vi "BPCS-Malicious-DE-OnePID.vi"() -> ()   [LabVIEW 2017]
uses:
  <vilib>/Platform/TimedLoop/XDataNode/timing_clust.ctl
  <vilib>/Platform/TimedLoop/XDataNode/nitl_modes.ctl
  <vilib>/Platform/TimedLoop/XDataNode/wakeup.ctl
  <vilib>/addons/control/pid/pid.llb/PID Advanced (DBL).vi
  <vilib>/Platform/TimedLoop/XDataNode/XDataNode.xnode
  <vilib>/Platform/TimedLoop/XDataNode/XDNodeRunTimeDep.lvlib
  <vilib>/addons/control/pid/NI_PID_pid.lvlib
panel:
  out "Finished Late? [i-1]":bool
  out "Actual End [i-1]":i64
  out "Expected End [i-1]":i64
  in  "stop":bool
  out "data out":string
  in  "Stop":bool
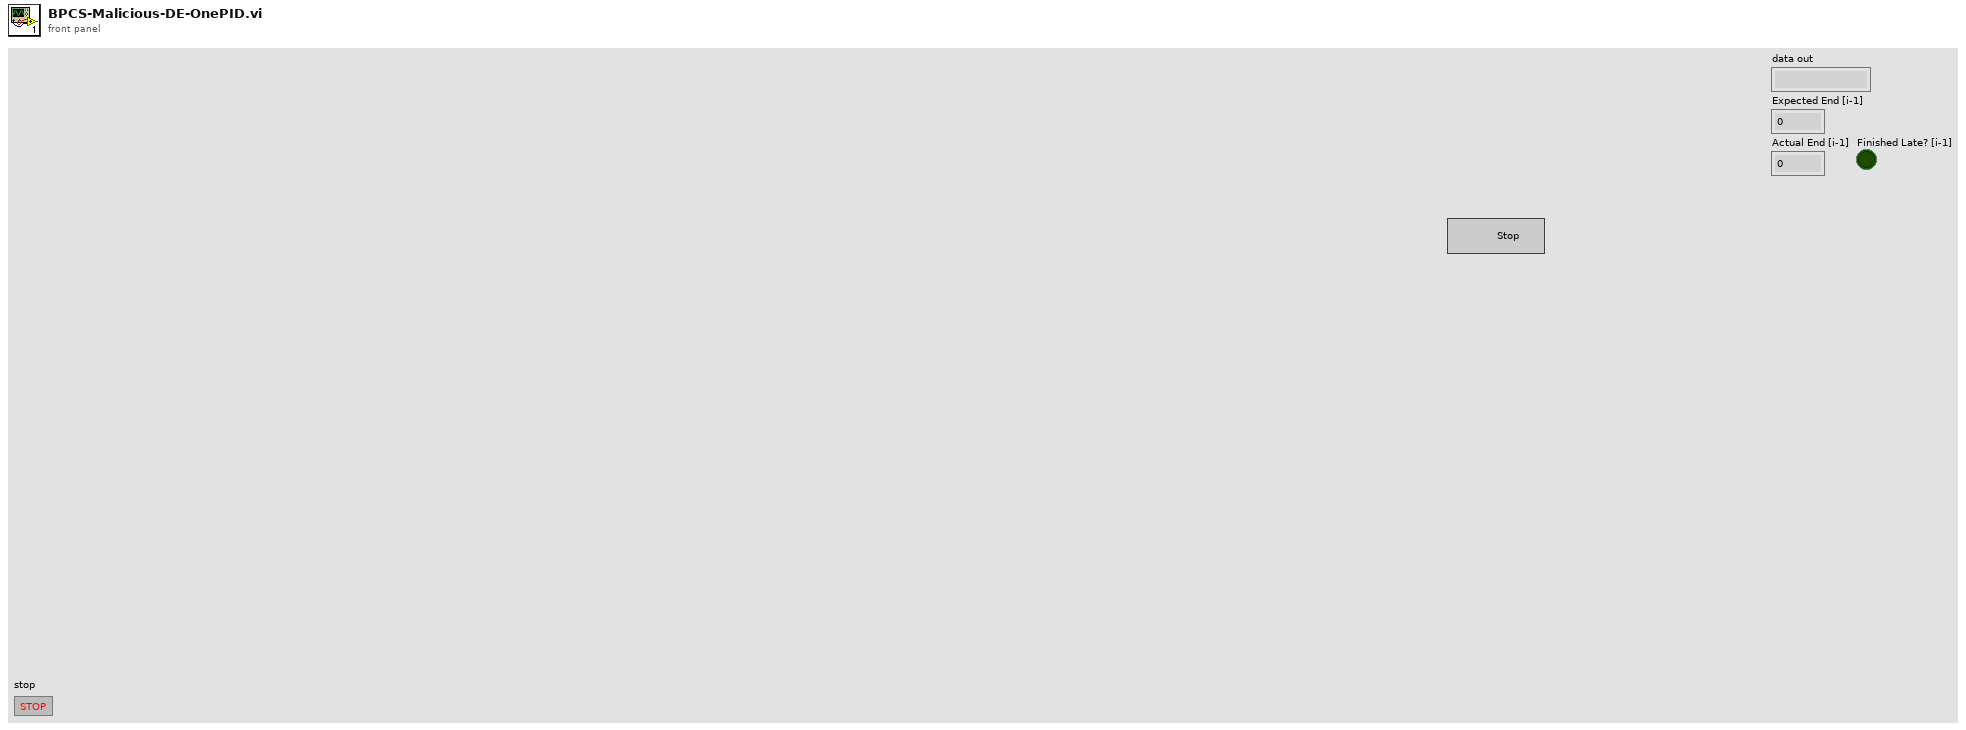
[diagram p1: front panel]
types:
  T1 = typedef "XDNodeRunTimeDep.lvlib/timing_clust.ctl" = cluster{"Expected End [f-1]":u64, "Actual End [f-1]":u64, "Finished Late? [f-1]":bool, "Expected End [i-1]":u64, "Actual End [i-1]":u64, "Finished Late? [i-1]":bool, "Expected Start [i]":u64, "Actual Start [i]":u64, "Expected Start [f]":u64, "Actual Start [f]":u64, "Source Name":string, "Structure Name":string, "Period":i64, "Deadline":i64, "Offset":i64, "Start":i64, "Priority":i32, "Timeout":i32, "Mode":T2, "Wakeup Reason":T3, "Error":errorcluster, "Source Type":string, "Secondary Source Type":string, "Global End Time":u64, "Global Start Time":u64, "Frame Duration":u64, "Iteration Duration":u64, "Assigned CPU":i32, "I/O Scan Engine Mode":u32}
  T2 = typedef "XDNodeRunTimeDep.lvlib/nitl_modes.ctl" = enum32{"No Change", "Process missed periods, maintain original phase", "Discard missed periods, maintain original phase", "Process missed periods, ignore original phase", "Discard missed periods, ignore original phase"}
  T3 = typedef "XDNodeRunTimeDep.lvlib/wakeup.ctl" = enum32{"Normal", "Aborted", "Asynchronous wakeup", "Timing source error", "Timed loop error", "Timeout"}
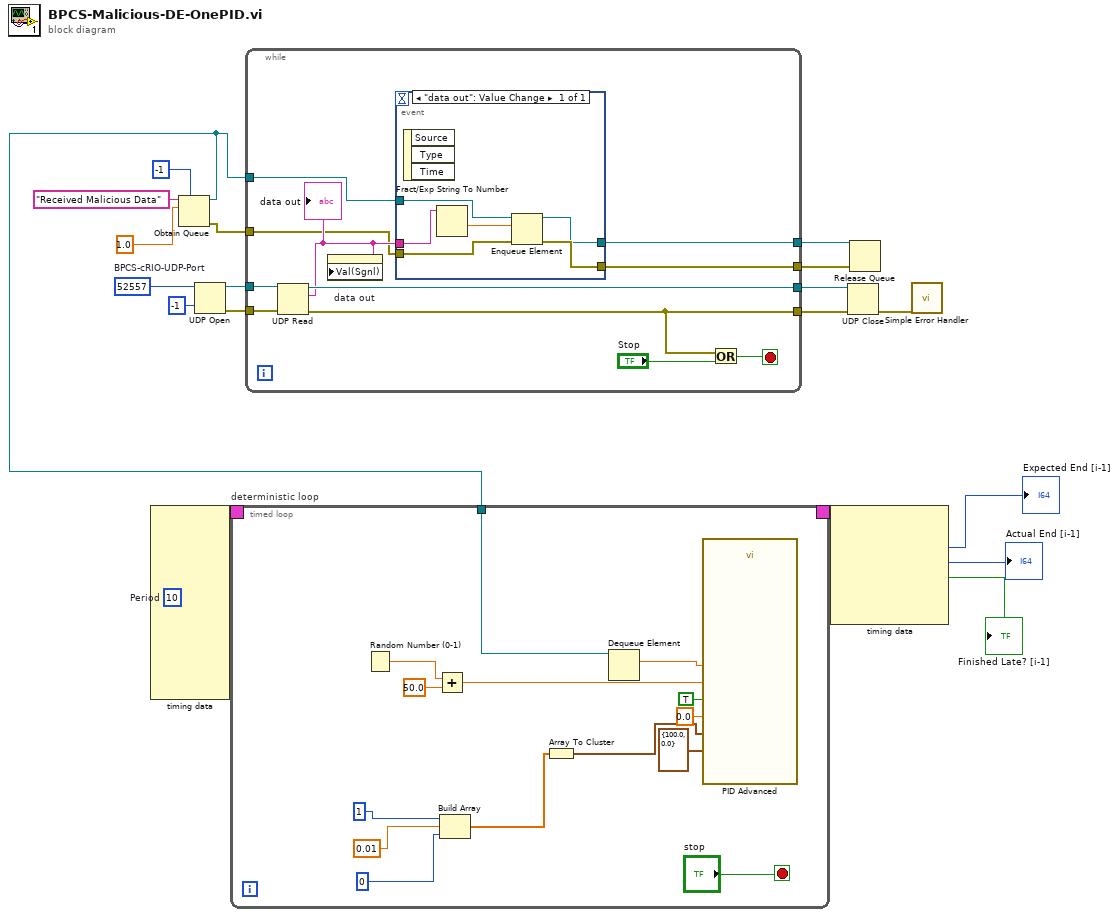
[diagram p0: block diagram]
diagram:
  w5 = i64 10  # Period
  w20 = u16 52557  # BPCS-cRIO-UDP-Port
  n1 = node-c288 ("Input Node")(w5) -> (w7:T1)  [unwired: 9 in]
  n2 = Obtain Queue(max queue size (-1, unlimited)=-1, name (unnamed)="Received Malicious Data", element data type=1.0) -> (queue out=w4:refnum<queue>, error out=w8:errorcluster)  [unwired: 2 in, 1 out]
  n3 = UDP Open(9:-1 ("timeout ms (25000)"), 11:w20) -> (port=w19:refnum<k16>, 0:w18:errorcluster)  [unwired: 3 in, 1 out]
  n4 = timed-loop "deterministic loop" {
    timing: w7 -> [_]
    timing-out: [_] -> w6
    tunnel: w4 -> [w32]
    stop <- "stop" stop-if-true
    n5 = Random Number (0-1)() -> (number: 0 to 1=w23:dbl)
    n6 = Add(x=w23, y=50.0) -> (x+y=w21:dbl)
    n7 = Build Array(1, 0.01, 0) -> (w27:dbl[])
    n8 = Array To Cluster(array=w27) -> (cluster=w26:cluster{"[0]":dbl, "[1]":dbl, "[2]":dbl})
    n9 = Dequeue Element(queue=w32) -> (element=w31:dbl)  [unwired: 2 in, 3 out]
    n10 = call-poly <vilib>:"PID Advanced.vi"("setpoint"=w31, "output range"=cluster{"output high":dbl, "output low":dbl} {"output high"=100.0, "output low"=0.0}, "auto? (T)"=TRUE, "manual control"=0.0, "process variable"=w21, "PID gains"=w26) -> ()  [unwired: 8 in, 2 out]
  }
  n11 = while {
    tunnel: w19 -> [w45]
    tunnel: w18 -> [w44]
    tunnel: [w43] -> w16
    tunnel: [w42] -> w15
    tunnel: [w41] -> w10
    tunnel: [w40] -> w9
    tunnel: w4 -> [w38]
    tunnel: w8 -> [w37]
    stop <- w46 stop-if-true
    n12 = UDP Read(connection ID=w45, 8:w44) -> (data out=w39:string, error out=w42:errorcluster, 3:w43:refnum<k16>)  [unwired: 1 in, 3 out]
    "data out" <- w39
    n13 = property on="data out" class="Str"("Val(Sgnl)"=w39) -> ()  [unwired: 2 in, 2 out]
    n14 = event shown="[0] \"data out\": Value Change" {
      selector: _ -> [_]
      dyn-events: _ -> [_]
      timeout: _ -> [_]
      tunnel: [w52] -> w41
      tunnel: [w51] -> w40
      tunnel: w39 -> [w50]
      tunnel: w38 -> [w49]
      tunnel: w37 -> [w48]
      event "data out": Value Change {
        n15 = event-data() -> ()  [unwired: 1 in, 3 out]
        n16 = Fract/Exp String To Number(string=w50) -> (number=w53:dbl)  [unwired: 3 in, 1 out]
        n17 = Enqueue Element(queue=w49, element=w53, error in (no error)=w48) -> (queue out=w51:refnum<queue>, error out=w52:errorcluster)  [unwired: 1 in, 1 out]
      }
    }
    n18 = Or(x=w42, y="Stop") -> (x .or. y?=w46:bool)
  }
  n19 = node-c288 ("Output Node")(w6) -> (→"Expected End [i-1]":i64, →"Actual End [i-1]":i64, →"Finished Late? [i-1]":bool)  [unwired: 3 out]
  n20 = UDP Close(connection ID=w16, 8:w15) -> (error out=w17:errorcluster)  [unwired: 1 out]
  n21 = Release Queue(queue=w9, error in (no error)=w10) -> ()  [unwired: 1 in, 3 out]
  n22 = call <vilib>:"Simple Error Handler.vi"("error in (no error)"=w17) -> ()  [unwired: 4 in, 5 out]
